vi "Read String A.vi"(8 "error in (no error)":errorcluster, 11 "One Terminal in":refnum<class "AbsFunc_One Term_STR.lvclass">) -> (0 "error out":errorcluster, 2 "Abs_String.lvclass":refnum<class "Abs_String.lvclass">, 3 "One Terminal out":refnum<class "AbsFunc_One Term_STR.lvclass">)   [LabVIEW 2021, in "AbsFunc_One Term_STR.lvclass"]
uses:
  AbsFunc_One Term_STR.lvclass
  Abs_Types/String/Abs_String.lvclass
  AbsFunc_One Term_STR.lvclass/AbsFunc_One Term_STR.ctl
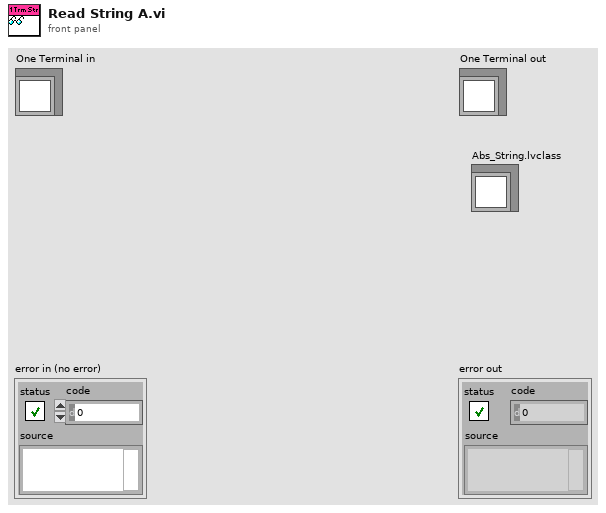
[diagram p1: front panel]
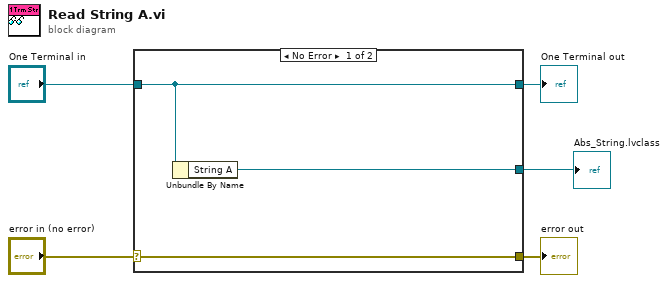
[diagram p0: block diagram]
diagram:
  n1 = case shown="No Error" "error in (no error)" {
    selector: "error in (no error)" -> [w8 w9]
    tunnel: [w8 w9] -> w4
    tunnel: [w7 w10] -> w2
    tunnel: "One Terminal in" -> [w7 w10]
    tunnel: [w6 _] -> w1
    frame No Error {
      n2 = Unbundle By Name(w7) -> ("String A"=w6:refnum<class "Abs_String.lvclass">)
    }
    frame Error {
    }
  }
  "error out" <- w4
  "One Terminal out" <- w2
  "Abs_String.lvclass" <- w1
